vi "Preset PART NUMBER query.vi"(8 "error in (no error)":errorcluster, 11 "VISA Refnum in":refnum<visa-resource-name>) -> (0 "error out":errorcluster, 2 "PART number":string, 3 "VISA Refnum out":refnum<visa-resource-name>)   [LabVIEW 2025, in "Chroma 19572.lvlib"]
uses:
  <vilib>/Utility/error.llb/Trim Whitespace One-Sided.vi
  <instrlib>/Chroma 19572/Chroma 19572.lvlib
panel:
  # "Set PART number query"
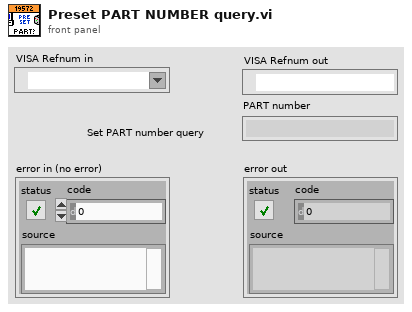
[diagram p1: front panel]
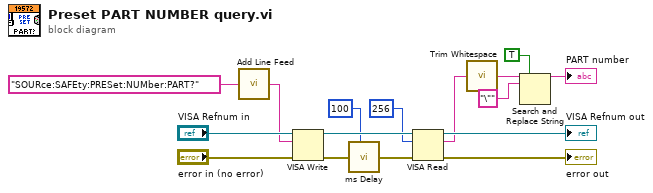
[diagram p0: block diagram]
diagram:
  n1 = call <instrlib>:"Add Line Feed.vi"("Command string"="SOURce:SAFEty:PRESet:NUMber:PART?") -> ("Concatenated string"=w8:string)  [unwired: 4 in]
  n2 = VISA Write(VISA resource name="VISA Refnum in", write buffer=w8, error in (no error)="error in (no error)") -> (VISA resource name out=w15:refnum<visa-resource-name>, error out=w14:errorcluster)  [unwired: 1 out]
  n3 = call <instrlib>:"ms Delay.vi"("miliseconds to wait"=u32 100 ("Time Delay ms"), "error in (no error)"=w14) -> ("error out"=w13:errorcluster)  [unwired: 6 in, 1 out]
  n4 = VISA Read(VISA resource name=w15, byte count=u32 256, error in (no error)=w13) -> (VISA resource name out=→"VISA Refnum out":refnum<visa-resource-name>, read buffer=w2:string, error out=→"error out":errorcluster)  [unwired: 1 out]
  n5 = call <vilib>:"Trim Whitespace.vi"("string"=w2) -> ("trimmed string"=w3:string)  [unwired: 1 in]
  n6 = Search and Replace String(replace all?=TRUE ("replace all? (F)"), input string=w3, search string="\"") -> (result string=→"PART number":string)  [unwired: 5 in, 3 out]
